vi "Sub_LEMP.vi"(0 "Eigen Values":dbl[](array[numeric]), 5 "Eigen Vectors":dbl[][](array[numeric]), 7 "STIFF Matrix":dbl[][](array[numeric]), 9 "Pin-Location":dbl, 11 "Mode Count":i32) -> (4 "Eigen Values Updated":dbl[](array[numeric]))   [LabVIEW 2019]
uses:
  Secular Solver/secular_solver.dll
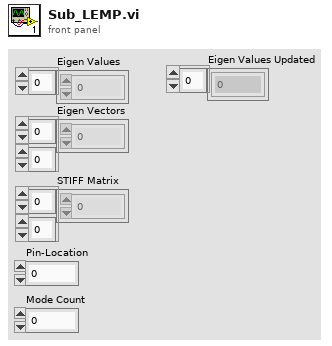
[diagram p1: front panel]
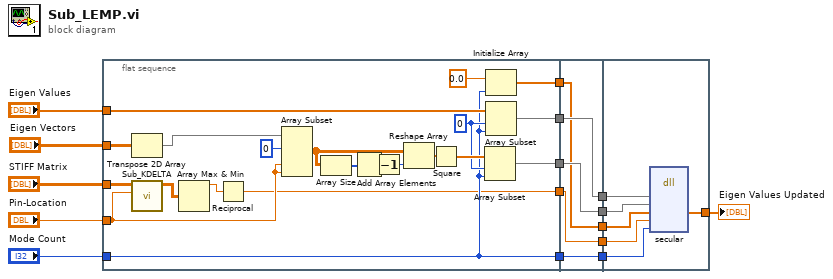
[diagram p0: block diagram]
diagram:
  n1 = flat-sequence {
    tunnel: "Eigen Vectors" -> [w37]
    tunnel: "STIFF Matrix" -> [w36]
    tunnel: "Pin-Location" -> [w31]
    tunnel: "Eigen Values" -> [w24]
    tunnel: "Mode Count" -> [w18]
    tunnel: [w21] -> w11
    tunnel: [w20] -> w10
    tunnel: [w19] -> w9
    tunnel: [w18] -> w8
    tunnel: [w17] -> w7
    tunnel: w11 -> [w40]
    tunnel: w10 -> [w42]
    tunnel: w9 -> [w41]
    tunnel: w8 -> [w38]
    tunnel: w7 -> [w39]
    tunnel: [w42] -> w6
    tunnel: [w41] -> w5
    tunnel: [w40] -> w4
    tunnel: [w39] -> w3
    tunnel: [w38] -> w2
    tunnel: w6 -> [w48]
    tunnel: w5 -> [w47]
    tunnel: w4 -> [w46]
    tunnel: w3 -> [w45]
    tunnel: w2 -> [w44]
    tunnel: [w43] -> w1
    frame #0 {
      w22 = 0 ("index")
      n2 = Transpose 2D Array(2D array=w37) -> (transposed array=w33:dbl[][])
      n3 = call "Sub_KDELTA.vi"("Pin-Location"=w31, "Pre-Pin Matrix"=w36) -> ("Pin-Delta Matrix"=w35:dbl[][])  [unwired: 8 in]
      n4 = Array Max & Min(array=w35) -> (max value=w34:dbl)  [unwired: 3 out]
      n5 = Reciprocal(x=w34) -> (1/x=w17:dbl)
      n6 = Array Subset(array=w33, index (row)=0 ("row 1"), index (col)=w31, length (col)=w31) -> (w27:dbl[][])  [unwired: 1 in]
      n7 = Array Size(array=w27) -> (size(s)=w30:i32[])
      n8 = Add Array Elements(numeric array=w30) -> (sum=w29:i32)
      n9 = Decrement(x=w29) -> (x-1=w28:i32)
      n10 = Reshape Array(w27, w28) -> (w26:dbl[])
      n11 = Square(x=w26) -> (x^2=w25:dbl[])
      n12 = Array Subset(array=w25, index=w22, length=w18) -> (w19:dbl[])
      n13 = Initialize Array(0.0 ("element"), w18) -> (w21:dbl[])
      n14 = Array Subset(array=w24, index=w22, length=w18) -> (w20:dbl[])
    }
    frame #1 {
    }
    frame #2 {
      n15 = dll-call lib="C:/Users/PXIe-8880/Documents/AFRL_summer_2022/LabVIEW_HIL/v0.2/Secular Solver/secular_solver.dll" fn="secular"("d"=w48, "v"=w47, "sol"=w46, "p"=w45, "mode"=w44) -> ("sol"=w43:dbl[])  [unwired: 8 in, 2 out]
    }
  }
  "Eigen Values Updated" <- w1
